vi "test11.vi"   [LabVIEW 2012]
uses:
  <vilib>/NXT/Block Support/NXT_InputPort.ctl
  <vilib>/NXT/Dual Mode Library/Display/drawNumber.vi
types:
  T1 = typedef "NXT_InputPort.ctl" = u8
  T2 = typedef "LVHSConnector.ctl" = cluster{"Hardware":string, "Flattened String":string}
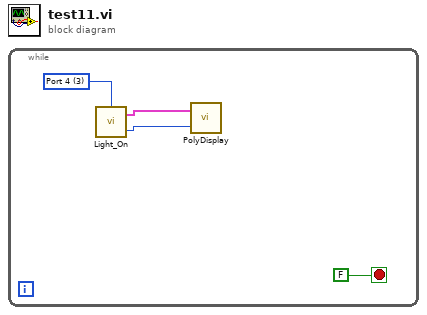
[diagram p0: block diagram]
diagram:
  n1 = while {
    stop <- FALSE stop-if-true
    w1 = T1 3 items=["Port 1", "Port 2", "Port 3", "Port 4"] ("Port (Port 3)")
    n2 = call <vilib>:"Light_On.vi"("Port (Port 3)"=w1) -> ("Scaled Value"=w4:i16, "NXT"=w3:T2)  [unwired: 2 in]
    n3 = call-poly <vilib>:"PolyDisplay.vi"("number"=w4, "NXT"=w3) -> ()  [unwired: 2 in, 1 out]
  }
